vi "Write Collimation data.vi"(7 "Send any changes now? (F)":bool, 8 "error in (no error)":errorcluster, 10 "BV Data":T1={"Centroid X[um]"=nan, "Centroid Y[um]"=nan, "PeakResp.[%]"=nan, "Knife Edge X[mm]"=nan, "Knife Edge Y[mm]"=nan, "Circularity"=nan, "Collimation Result"=FALSE} {"PeakResp.[%]" format="%.0g"}, 11 "Fiber Auto Collimation state data in":refnum<class "Fiber Auto Collimation state data.lvclass">) -> (0 "error out":errorcluster, 3 "Fiber Auto Collimation state data out":refnum<class "Fiber Auto Collimation state data.lvclass">)   [LabVIEW 2018, in "Fiber Auto Collimation state data.lvclass"]
uses:
  Fiber Auto Collimation state data.lvclass
  BV Data.ctl
  Tracked state data.ctl
  Fiber Auto Collimation state data.lvclass/Fiber Auto Collimation state data.ctl
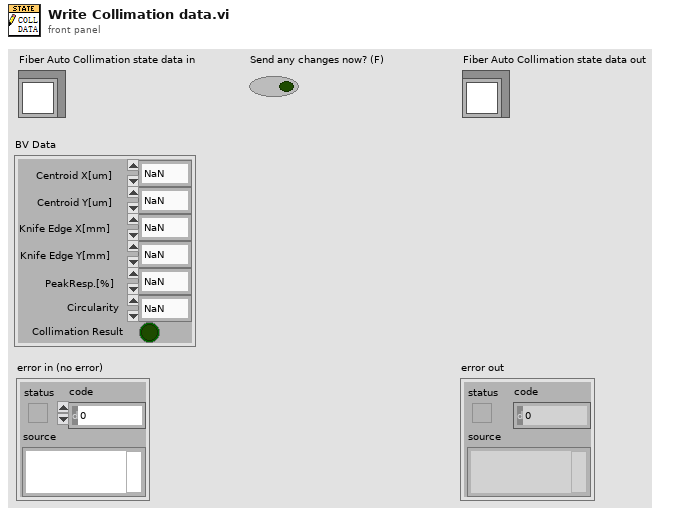
[diagram p1: front panel]
types:
  T1 = typedef "Fiber Auto Collimation state data.lvclass/BV Data.ctl" = cluster{"Centroid X[um]":sgl, "Centroid Y[um]":sgl, "PeakResp.[%]":dbl, "Knife Edge X[mm]":sgl, "Knife Edge Y[mm]":sgl, "Circularity":sgl, "Collimation Result":bool}
  T2 = typedef "Fiber Auto Collimation state data.lvclass/Tracked state data.ctl" = enum16{"No update", "Permission level", "Username", "Test running", "DUT Serial", "Test status", "MOM Lot", "Loaded test recipe", "Model case running", "Station status", "BV data", "Defect Identify data", "Axis Position data", "Fiber Ass PN", "Operator", "RunTime", "VBAI", "Steps Cycle Time"}
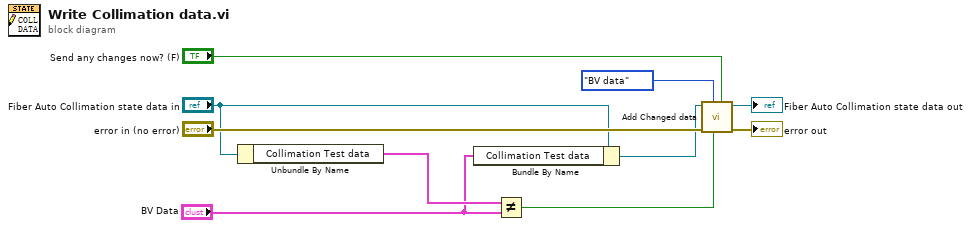
[diagram p0: block diagram]
diagram:
  n1 = Unbundle By Name("Fiber Auto Collimation state data in") -> ("Collimation Test data"=w3:T1)
  n2 = Bundle By Name(cluster="Fiber Auto Collimation state data in", "Collimation Test data"="BV Data") -> (w7:refnum<class "Fiber Auto Collimation state data.lvclass">)
  n3 = Not Equal?(x=w3, y="BV Data") -> (x != y?=w4:bool)
  n4 = call "Add Changed data.vi"("Send any changes now? (F)"="Send any changes now? (F)", "Data changed?"=w4, "Data type"=Tracked_state_data."BV data", "error in (no error)"="error in (no error)", "Fiber Auto Collimation state data in"=w7) -> ("error out"=→"error out":errorcluster, "Fiber Auto Collimation state data out"=→"Fiber Auto Collimation state data out":refnum<class "Fiber Auto Collimation state data.lvclass">)  [unwired: 5 in]
